vi "Lectura en PEM.vi"(0 "Caracteristica a leer":u16(ring) items=["Retardo", "Longitud de onda", "Frecuencia 1", "Frecuencia 2"], 1 "VISA resource name":refnum<visa-resource-name>, 2 "error in (no error)":errorcluster) -> (3 "Valor leído":dbl, 4 "Magnitud":u16(ring) items=["Lambda", "nm", "Hz", "Hz"], 5 "VISA resource name out":refnum<visa-resource-name>, 6 "error out":errorcluster)   [LabVIEW 2018]
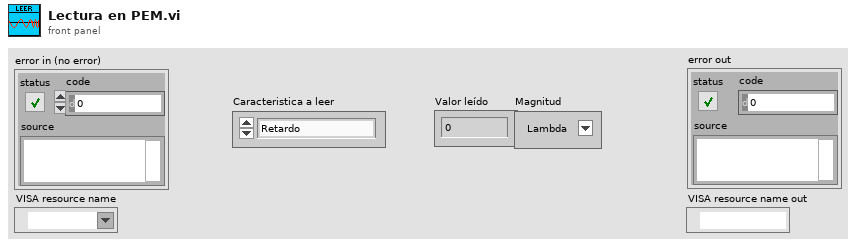
[diagram p1: front panel]
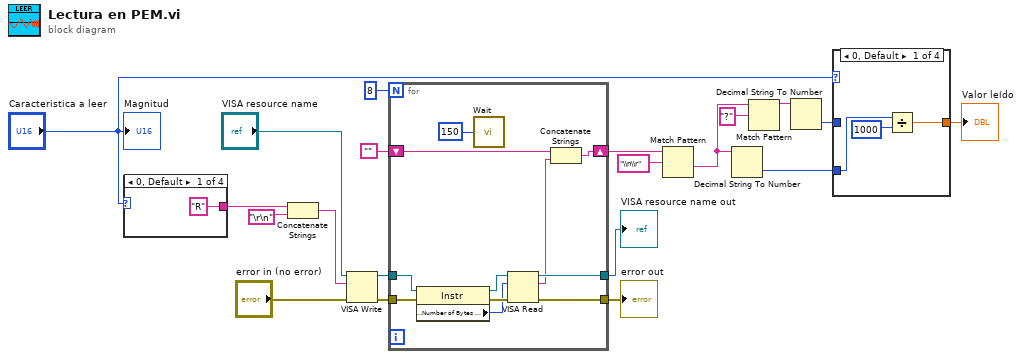
[diagram p0: block diagram]
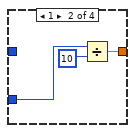
[diagram p2: hidden frame]
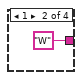
[diagram p5: hidden frame]
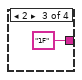
[diagram p6: hidden frame]
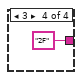
[diagram p7: hidden frame]
diagram:
  n1 = case shown="0, Default" "Caracteristica a leer" {
    tunnel: ["R" ("string") "W" ("string") "1F" ("string") "2F" ("string")] -> w11
    frame 0, Default {
    }
    frame 1 {
    }
    frame 2 {
    }
    frame 3 {
    }
  }
  n2 = Concatenate Strings(w11, "\r\n") -> (w18:string)
  n3 = VISA Write(VISA resource name="VISA resource name", write buffer=w18, error in (no error)="error in (no error)") -> (VISA resource name out=w16:refnum<visa-resource-name>, error out=w15:errorcluster)  [unwired: 1 out]
  n4 = for {
    N: 8 -> [_]
    tunnel: [w35] -> w3
    tunnel: w16 -> [w34]
    tunnel: w15 -> [w33]
    tunnel: [w30] -> w14
    shift-right: [w28] -> w12
    shift-left: "" -> [w25]
    n5 = property class="Instr"(reference=w34, error in=w33) -> (reference out=w32:refnum<visa-resource-name>, error out=w31:errorcluster, "Serial Settings:Number of Bytes at Serial Port"=w27:u32)
    n6 = call "Wait"("Count(mSec)"=u32 150) -> ()  [unwired: 1 out]
    n7 = VISA Read(VISA resource name=w32, byte count=w27, error in (no error)=w31) -> (VISA resource name out=w35:refnum<visa-resource-name>, read buffer=w29:string, error out=w30:errorcluster)  [unwired: 1 out]
    n8 = Concatenate Strings(w25, w29) -> (w28:string)
  }
  "VISA resource name out" <- w3
  "error out" <- w14
  n9 = Match Pattern(string=w12, regular expression="\\n\\r") -> (after substring=w9:string)  [unwired: 1 in, 3 out]
  n10 = Decimal String To Number(string=w9) -> (number=w7:i32)  [unwired: 2 in, 1 out]
  n11 = Match Pattern(string=w9, regular expression="?") -> (before substring=w6:string)  [unwired: 1 in, 3 out]
  n12 = Decimal String To Number(string=w6) -> (number=w5:i32)  [unwired: 2 in, 1 out]
  n13 = case shown="0, Default" "Caracteristica a leer" {
    tunnel: w7 -> [w38 w39 _ _]
    tunnel: [w37 w40 w42 w43] -> w10
    tunnel: w5 -> [_ _ w42 w43]
    frame 0, Default {
      n14 = Divide(x=w38, y=1000) -> (x/y=w37:dbl)
    }
    frame 1 {
      n15 = Divide(x=w39, y=10) -> (x/y=w40:dbl)
    }
    frame 2 {
    }
    frame 3 {
    }
  }
  "Valor leído" <- w10
  "Magnitud" <- "Caracteristica a leer"
